vi "ALTS-2015 Simulate Write Result DB.vi"(8 "error in":errorcluster, 10 "Options":T1, 11 "Simulate Result DB Path":path) -> (0 "error out":errorcluster)   [LabVIEW 2013]
uses:
  Controls/ALTS-2015 write DB Result cases.ctl
  <vilib>/Utility/file.llb/Write To Spreadsheet File (string).vi
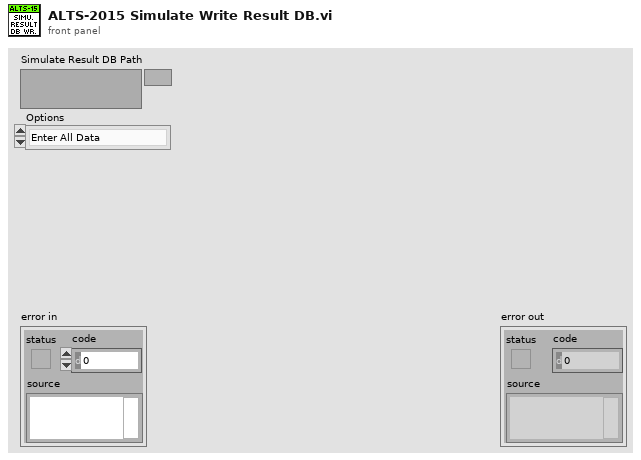
[diagram p1: front panel]
types:
  T1 = typedef "ALTS-2015 write DB Result cases.ctl" = enum16{"Enter All Data", "Enter WO & SN"}
  T2 = typedef "ALTS-2015 DB Result Cluster.ctl" = cluster{"Sensor_Name":string, "SN":string, "Work_order_Number":string, "User1":string, "User2":string, "User3":string, "User4":string, "Pressure":dbl, "Flow":dbl, "Test_Result":string, "Test_Time":string}
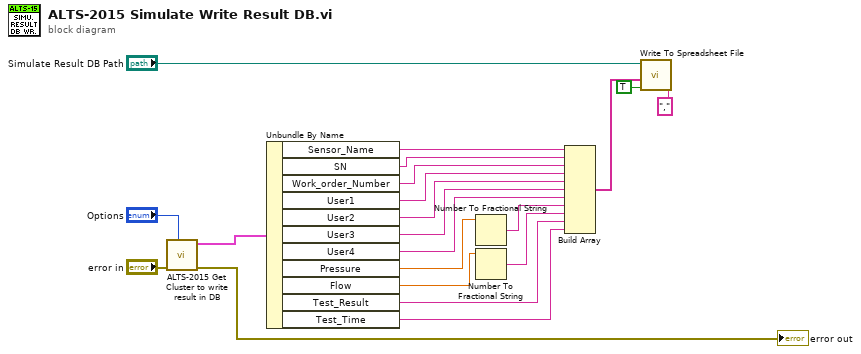
[diagram p0: block diagram]
diagram:
  n1 = call "ALTS-2015 Get Cluster to write result in DB.vi"("Options"="Options", "error in"="error in") -> ("error out"=→"error out":errorcluster, "DB Result Cluster Out"=w20:T2)  [unwired: 8 in]
  n2 = Unbundle By Name(w20) -> ("Sensor_Name"=w3:string, "SN"=w15:string, "Work_order_Number"=w14:string, "User1"=w13:string, "User2"=w12:string, "User3"=w11:string, "User4"=w10:string, "Pressure"=w17:dbl, "Flow"=w16:dbl, "Test_Result"=w7:string, "Test_Time"=w6:string)
  n3 = Number To Fractional String(number=w17) -> (F-format string=w9:string)  [unwired: 3 in]
  n4 = Number To Fractional String(number=w16) -> (F-format string=w8:string)  [unwired: 3 in]
  n5 = Build Array(w3, w15, w14, w13, w12, w11, w10, w9, w8, w7, w6) -> (w5:string[])
  n6 = call-poly <vilib>:"Write To Spreadsheet File.vi"("delimiter (\\t)"="," ("delimiter (\\t)"), "append to file? (new file:F)"=TRUE, "1D data"=w5, "file path (dialog if empty)"="Simulate Result DB Path") -> ()  [unwired: 4 in, 1 out]
